vi "initialInternalConf.vi"(8 "error in (no error)":errorcluster, 11 "ElectrometerInternalConfiguration in":refnum<class "ElectrometerInternalConfiguration.lvclass">) -> (0 "error out":errorcluster, 3 "ElectrometerInternalConfiguration out":refnum<class "ElectrometerInternalConfiguration.lvclass">)   [LabVIEW 2016, in "ElectrometerInternalConfiguration.lvclass"]
uses:
  ElectrometerInternalConfiguration.lvclass
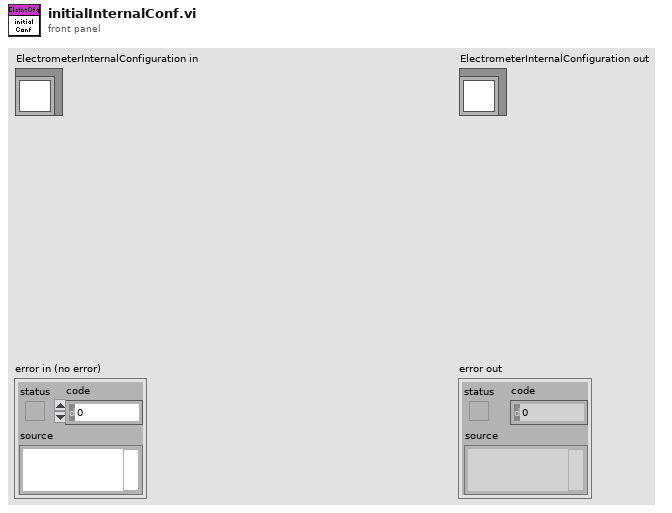
[diagram p1: front panel]
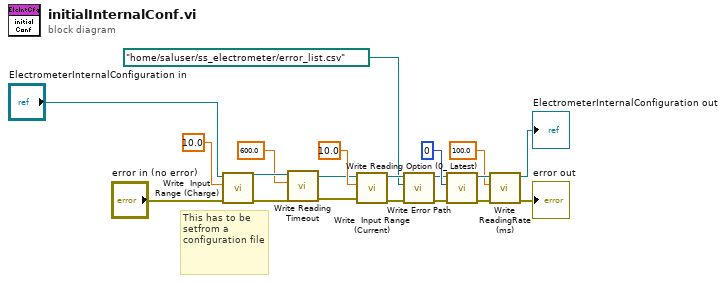
[diagram p0: block diagram]
diagram:
  # "This has to be setfrom a configuration file"
  n1 = call-dynamic "Write  Input Range (Charge).vi"("error in (no error)"="error in (no error)", "Input Range (Charge)"=10.0, "ElectrometerInternalConfiguration in"="ElectrometerInternalConfiguration in") -> ("error out"=w5:errorcluster, "ElectrometerInternalConfiguration out"=w2:refnum<class "ElectrometerInternalConfiguration.lvclass">)  [unwired: 7 in]
  n2 = call-dynamic "Write Reading Timeout.vi"("error in (no error)"=w5, "Reading Timeout"=600.0, "ElectrometerInternalConfiguration in"=w2) -> ("error out"=w4:errorcluster, "ElectrometerInternalConfiguration out"=w3:refnum<class "ElectrometerInternalConfiguration.lvclass">)  [unwired: 7 in]
  n3 = call-dynamic "Write  Input Range (Current).vi"("error in (no error)"=w4, "Input Range (Current)"=10.0, "ElectrometerInternalConfiguration in"=w3) -> ("error out"=w10:errorcluster, "ElectrometerInternalConfiguration out"=w7:refnum<class "ElectrometerInternalConfiguration.lvclass">)  [unwired: 7 in]
  n4 = call-dynamic "Write Error Path.vi"("error in (no error)"=w10, "Error Path"=path "/home/saluser/ss_electrometer/error_list.csv", "ElectrometerInternalConfiguration in"=w7) -> ("error out"=w9:errorcluster, "ElectrometerInternalConfiguration out"=w8:refnum<class "ElectrometerInternalConfiguration.lvclass">)  [unwired: 7 in]
  n5 = call-dynamic "Write Reading Option (0_ Latest).vi"("error in (no error)"=w9, "Reading Option (0: Latest)"=0, "ElectrometerInternalConfiguration in"=w8) -> ("error out"=w16:errorcluster, "ElectrometerInternalConfiguration out"=w19:refnum<class "ElectrometerInternalConfiguration.lvclass">)  [unwired: 7 in]
  n6 = call-dynamic "Write ReadingRate (ms).vi"("error in (no error)"=w16, "ReadingRate (ms)"=100.0, "ElectrometerInternalConfiguration in"=w19) -> ("error out"=→"error out":errorcluster, "ElectrometerInternalConfiguration out"=→"ElectrometerInternalConfiguration out":refnum<class "ElectrometerInternalConfiguration.lvclass">)  [unwired: 7 in]
